vi "CenterFinder.vi"() -> ()   [LabVIEW 2016]
uses:
  Control/ProcessCtl.ctl
  <vilib>/userdefined/High Color/IMAQdx.ctl
  <vilib>/vision/driver/NI_Vision_Acquisition_Software.lvlib
  <vilib>/vision/NI_Vision_Development_Module.lvlib
panel:
  out "Array":T1(array[cluster])
  out "output cluster":cluster{"X":dbl, "Y":dbl, "Z":dbl}
  out "1":bool[](array[boolean])
  in  "Enum":enum16{"B2T", "L2R", "R2L", "T2B"}(ring)=enum."R2L"
  in  "Delete":bool
  in  "Retake":bool
  in  "Next":bool
  in  "Process":bool
  in  "Acquire":bool
  in  "stop":bool
  out "Image":T2(plugin-control)
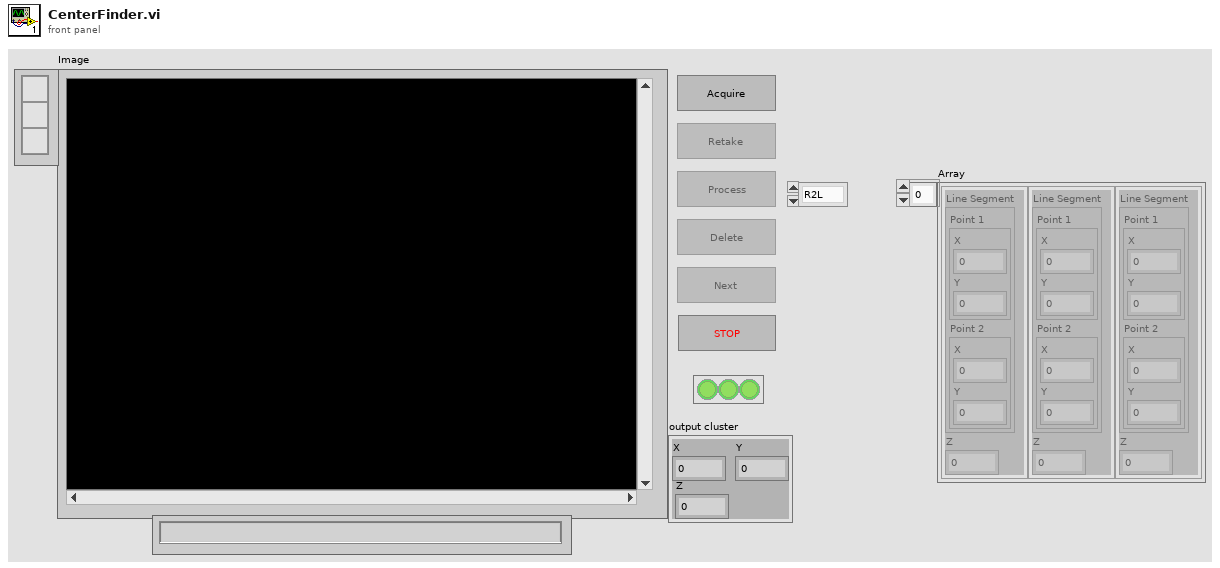
[diagram p1: front panel]
types:
  T1 = cluster{"Line Segment":cluster{"Point 1":cluster{"X":sgl, "Y":sgl}, "Point 2":cluster{"X":sgl, "Y":sgl}}, "Z":dbl}[]
  T2 = typedef "IMAQ Image.ctl" = refnum<image>
  T3 = typedef "IMAQdx.ctl" = refnum<k21>
  T4 = typedef "ProcessCtl.ctl" = enum16{"Idle", "Acquire", "Process", "Abort", "Initialize", "Wait"}
  T5 = enum8{"Enabled", "Disabled", "Disabled and Grayed Out"}
  T6 = cluster{"Line Segment":cluster{"Point 1":cluster{"X":sgl, "Y":sgl}, "Point 2":cluster{"X":sgl, "Y":sgl}}, "Z":dbl}
  T7 = cluster{"Edge Polarity":u16, "Kernel Size":u32, "Width":u32, "Minimum Edge Strength":dbl, "Interpolation Type":u16, "Data Processing Method":u16}
  T8 = typedef "Image Type" = u32
  T9 = typedef "IMAQ Line" = cluster{"Start X":i32, "Start Y":i32, "End X":i32, "End Y":i32}
  T10 = typedef "ROI Descriptor" = cluster{"Global Rectangle":i32[], "Contours":cluster{"ID":enum32{"External", "Internal"}, "Type":u32, "Coordinates":i32[]}[]}
  T11 = typedef "Edge New.ctl" = cluster{"Location (Pixel)":cluster{"X":sgl, "Y":sgl}, "Location (Real-World)":cluster{"X":sgl, "Y":sgl}, "Distance (Pixel)":dbl, "Distance (Real-World)":dbl, "Strength":dbl, "Noise":dbl, "Rising?":bool}
  T12 = cluster{"Point 1":cluster{"X":sgl, "Y":sgl}, "Point 2":cluster{"X":sgl, "Y":sgl}}
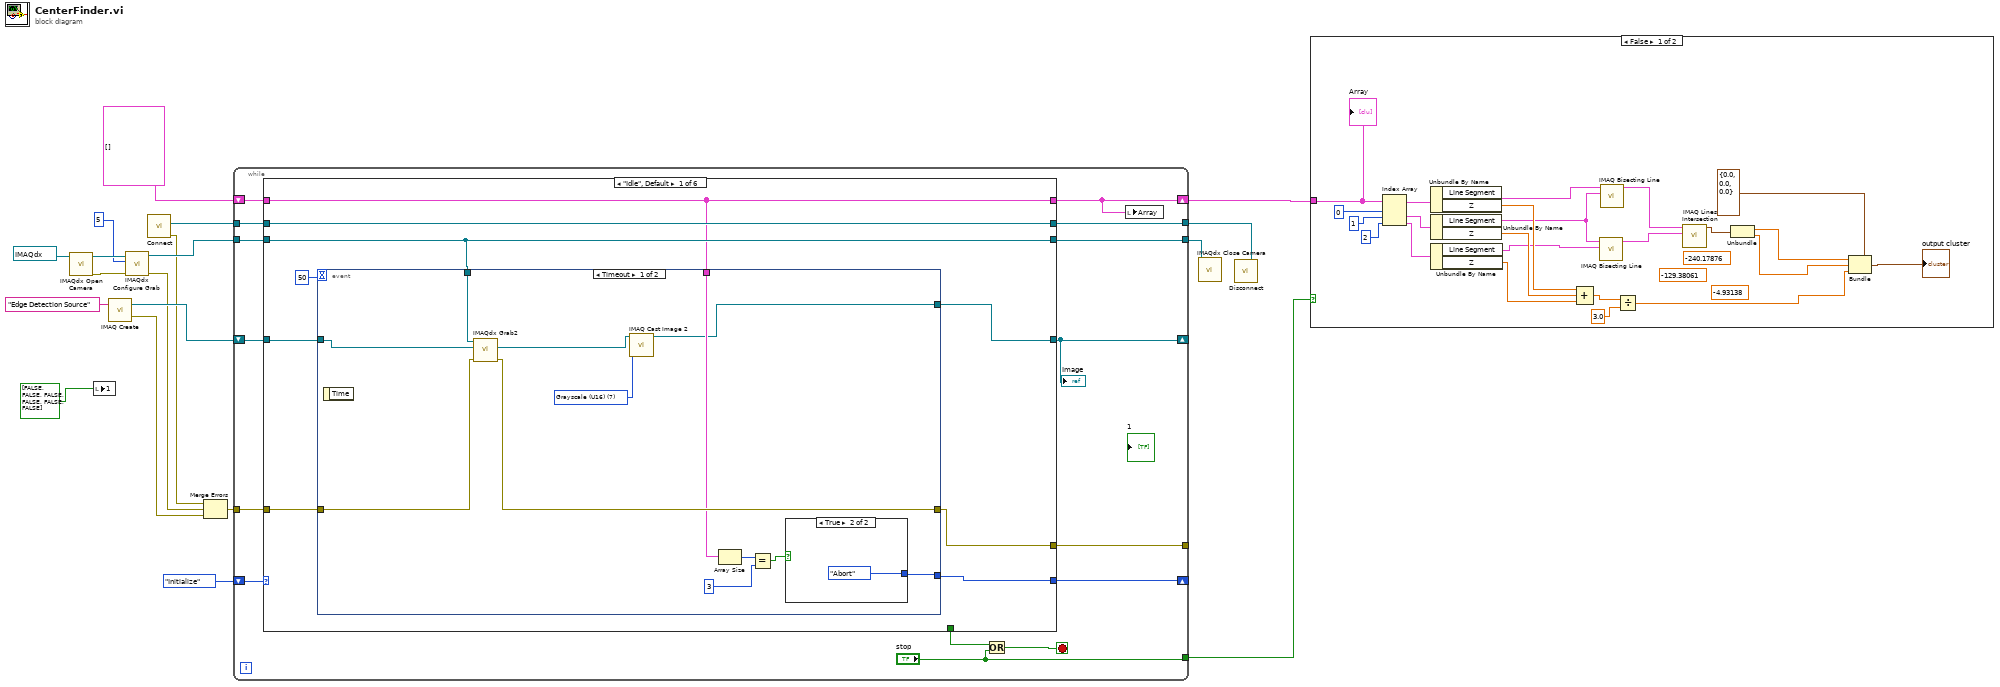
[diagram p0: block diagram]
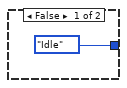
[diagram p3: hidden frame]
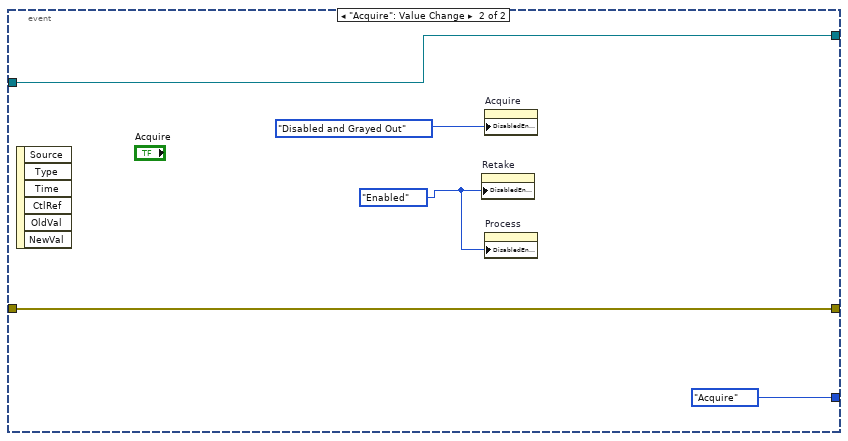
[diagram p4: hidden frame]
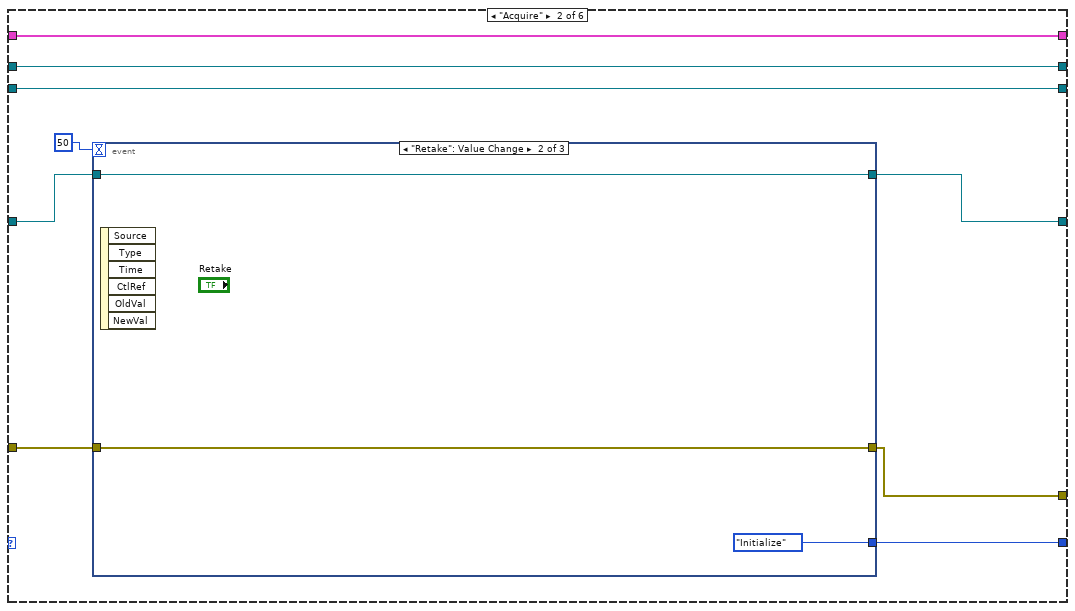
[diagram p5: hidden frame]
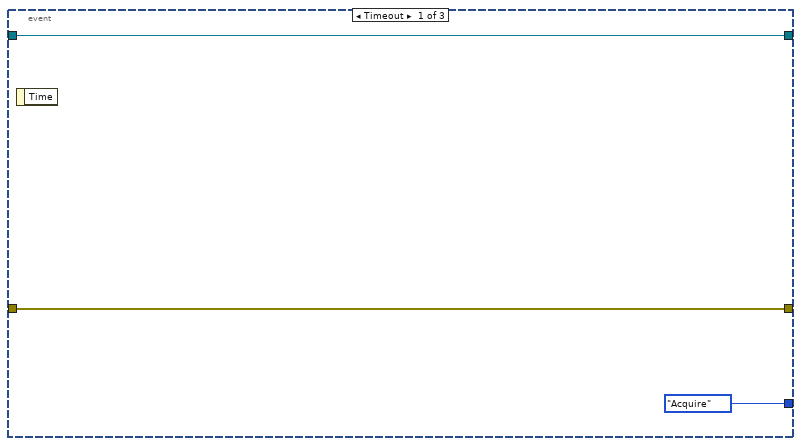
[diagram p6: hidden frame]
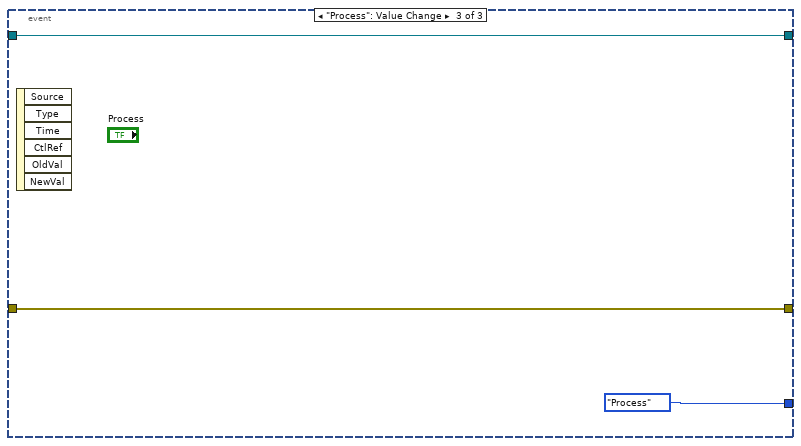
[diagram p7: hidden frame]
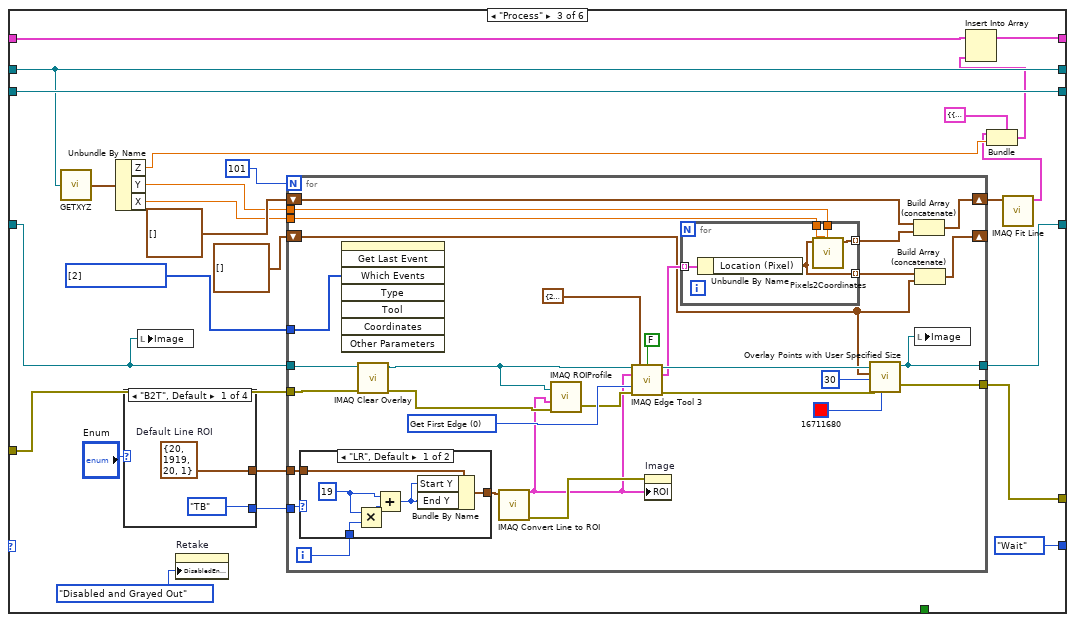
[diagram p8: hidden frame]
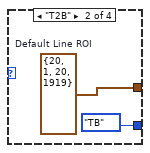
[diagram p9: hidden frame]
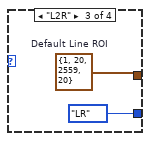
[diagram p10: hidden frame]
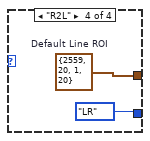
[diagram p11: hidden frame]
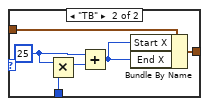
[diagram p12: hidden frame]
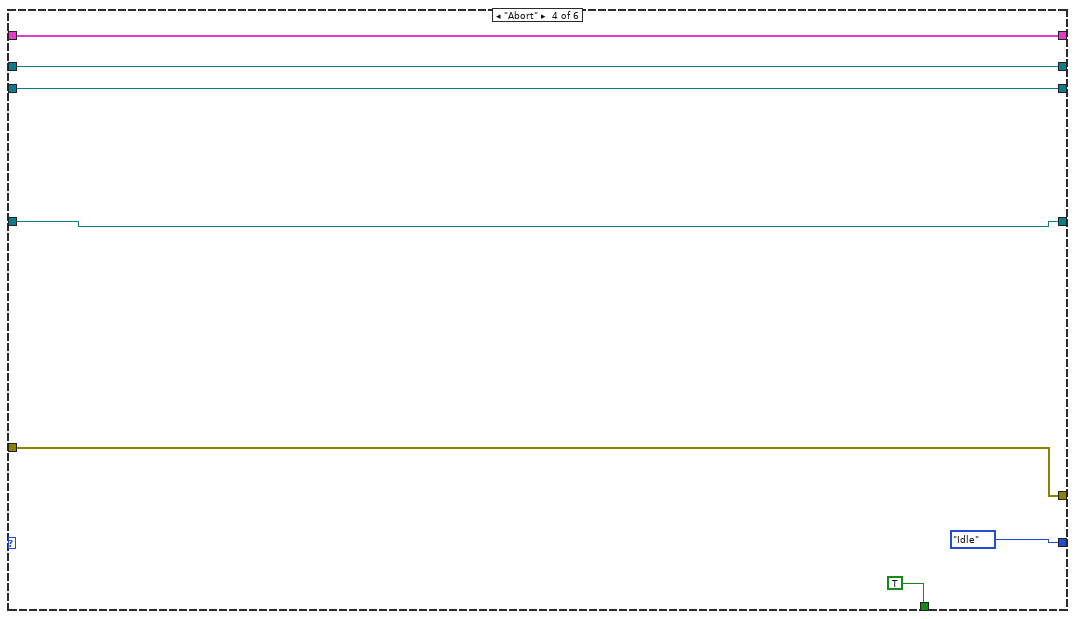
[diagram p13: hidden frame]
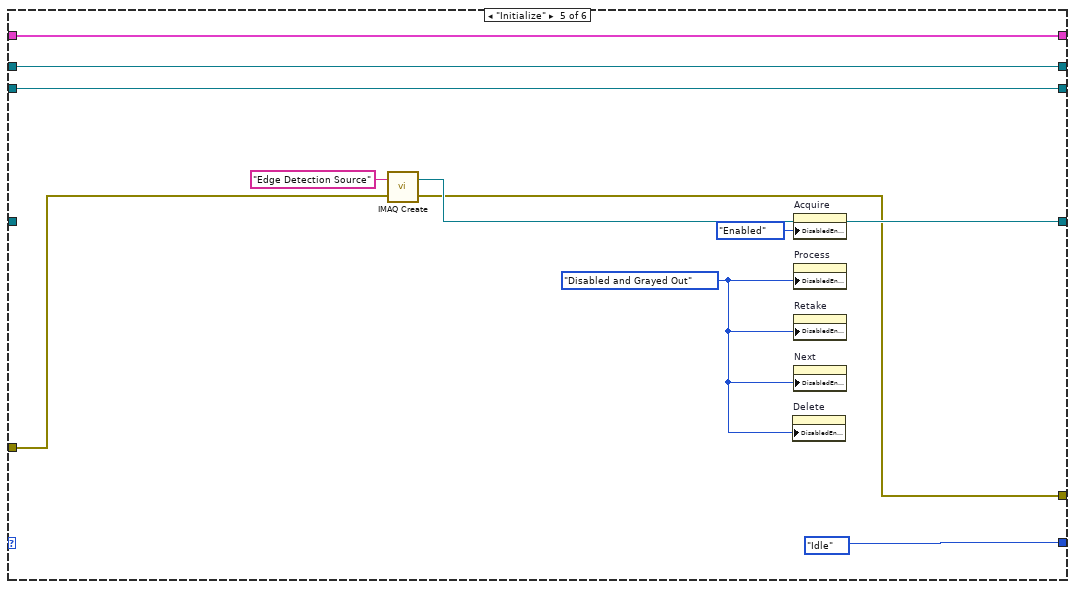
[diagram p14: hidden frame]
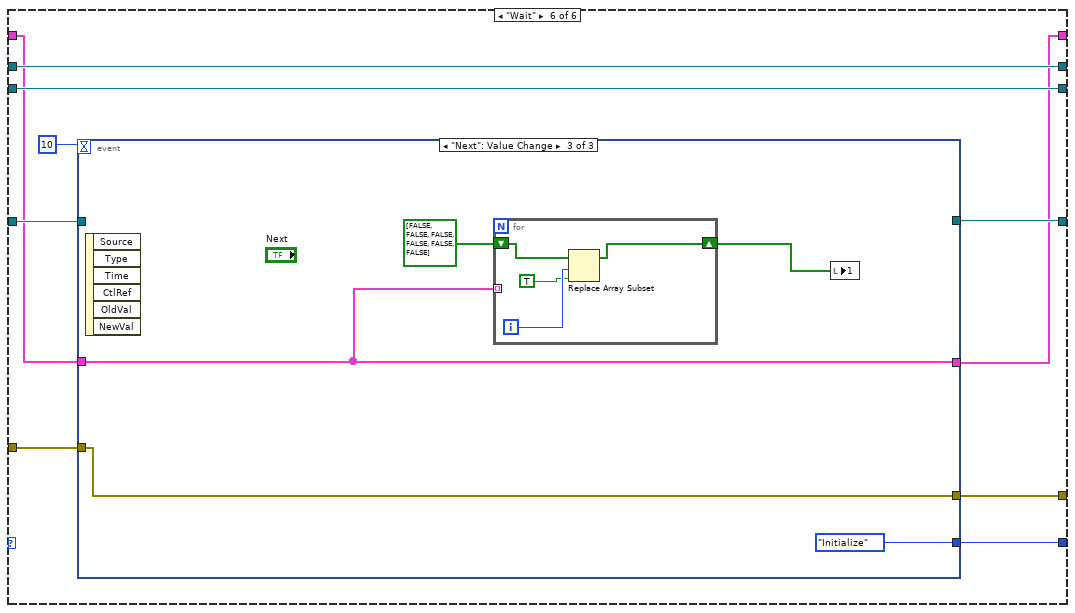
[diagram p15: hidden frame]
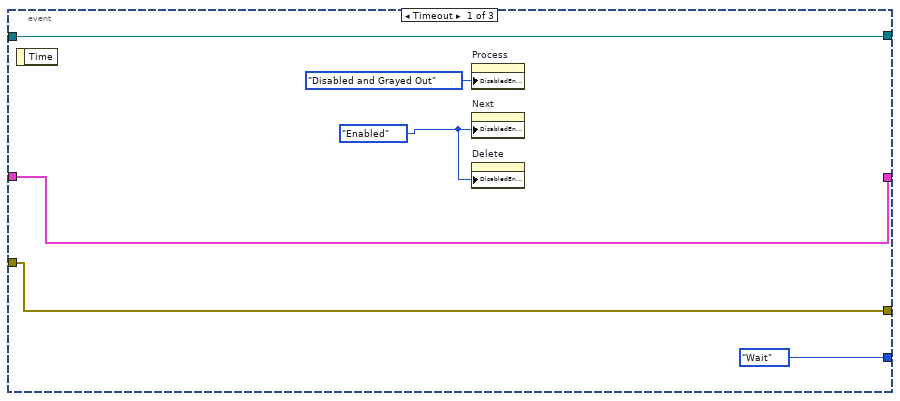
[diagram p16: hidden frame]
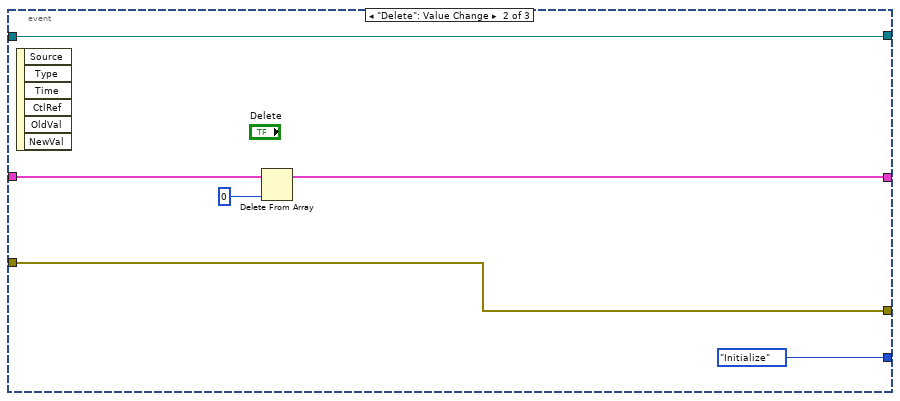
[diagram p17: hidden frame]
diagram:
  n1 = call <vilib>:"IMAQdx Open Camera.vi"("Session In"=T3 "cam0") -> ("error out"=w16:errorcluster, "Session Out"=w17:T3)  [unwired: 9 in]
  n2 = local write "1"(bool[] [FALSE, FALSE, FALSE, FALSE, FALSE, FALSE] ("1 2")) -> ()
  n3 = call "IMAQ Create"("Image Name"="Edge Detection Source") -> ("New Image"=w14:T2, "error out"=w7:errorcluster)  [unwired: 4 in]
  n4 = call <vilib>:"IMAQdx Configure Grab.vi"("error in"=w16, "Number of Buffers"=u32 5, "Session In"=w17) -> ("error out"=w8:errorcluster, "Session Out"=w18:T3)  [unwired: 7 in]
  n5 = call "Connect.vi"() -> ("error out"=w9:errorcluster, "controller"=w11:refnum<k24>)  [unwired: 10 in]
  n6 = Merge Errors(w9, w8, w7) -> (w6:errorcluster)
  n7 = while {
    tunnel: w18 -> [w25]
    tunnel: [w24] -> w12
    shift-right: [w31] -> _
    shift-left: w14 -> [w29]
    tunnel: w11 -> [w27]
    tunnel: [w26] -> w10
    tunnel: w6 -> [w34]
    shift-right: [w32] -> _
    shift-left: ProcessCtl."Initialize" -> [w33]
    tunnel: [w30] -> _
    shift-right: [w21] -> w2
    shift-left: T1 [] -> [w28]
    tunnel: ["stop"] -> w1
    stop <- w22 stop-if-true
    n8 = case shown="\"Idle\", Default" w33 {
      tunnel: w34 -> [w43 w67 w104 w161 w173 w179]
      tunnel: [w39 w68 ProcessCtl."Wait" ProcessCtl."Idle" ProcessCtl."Idle" w185] -> w32
      tunnel: w29 -> [w42 w71 w86 w164 _ w187]
      tunnel: [w41 w70 w96 w164 w174 w186] -> w31
      tunnel: [w38 w66 w90 w161 w172 w180] -> w30
      tunnel: w28 -> [w35 w65 w92 w167 w171 w182]
      tunnel: [w35 w65 w91 w167 w171 w181] -> w21
      tunnel: w27 -> [w37 w64 w93 w166 w170 w184]
      tunnel: [w37 w64 w93 w166 w170 w184] -> w26
      tunnel: w25 -> [w36 w63 w94 w165 w169 w183]
      tunnel: [w36 w63 w94 w165 w169 w183] -> w24
      tunnel: [_ _ _ TRUE _ _] -> w23
      frame "Idle", Default {
        n9 = event shown="[0] Timeout" {
          selector: _ -> [_ _]
          dyn-events: _ -> [_ _]
          timeout: 50 -> [_ _]
          tunnel: w43 -> [w55 w58]
          tunnel: w42 -> [w54 w60]
          tunnel: w36 -> [w53 _]
          tunnel: [w45 w60] -> w41
          tunnel: [w51 ProcessCtl."Acquire"] -> w39
          tunnel: [w52 w58] -> w38
          tunnel: w35 -> [w50 _]
          event Timeout {
            w46 = T8 7 items=["Grayscale (U8)", "Grayscale (I16)", "Grayscale (SGL)", "Complex (CSG)", "RGB (U32)", "HSL (U32)", "RGB (U64)", "Grayscale (U16)"] ("Image Type")
            n10 = event-data() -> ()  [unwired: 1 in, 1 out]
            n11 = call <vilib>:"IMAQdx Grab2.vi"("error in"=w55, "Image In"=w54, "Session In"=w53) -> ("error out"=w52:errorcluster, "Image Out"=w44:T2)  [unwired: 5 in, 2 out]
            n12 = call "IMAQ Cast Image 2"("Image Src"=w44, "Image Type"=w46) -> ("Image Dst Out"=w45:T2)  [unwired: 12 in, 1 out]
            n13 = Array Size(array=w50) -> (size(s)=w49:i32)
            n14 = Equal?(x=w49, y=3) -> (x = y?=w47:bool)
            n15 = case shown="True" w47 {
              tunnel: [ProcessCtl."Idle" ProcessCtl."Abort"] -> w51
              frame False {
              }
              frame True {
              }
            }
          }
          event "Acquire": Value Change {
            w59 = T5."Enabled" ("Disabled")
            n16 = event-data() -> ()  [unwired: 1 in, 6 out]
            n17 = property on="Retake" class="Bool"("DisabledEnum"=w59) -> ()  [unwired: 2 in, 2 out]
            n18 = property on="Acquire" class="Bool"("DisabledEnum"=T5."Disabled and Grayed Out" ("Disabled")) -> ()  [unwired: 2 in, 2 out]
            n19 = property on="Process" class="Bool"("DisabledEnum"=w59) -> ()  [unwired: 2 in, 2 out]
          }
        }
      }
      frame "Acquire" {
        n20 = event shown="[1] \"Retake\": Value Change" {
          selector: _ -> [_ _ _]
          dyn-events: _ -> [_ _ _]
          timeout: 50 -> [_ _ _]
          tunnel: w71 -> [w74 w75 w78]
          tunnel: [w74 w75 w78] -> w70
          tunnel: [ProcessCtl."Acquire" ProcessCtl."Initialize" ProcessCtl."Process"] -> w68
          tunnel: w67 -> [w72 w76 w79]
          tunnel: [w72 w76 w79] -> w66
          event Timeout {
            n21 = event-data() -> ()  [unwired: 1 in, 1 out]
          }
          event "Retake": Value Change {
            n22 = event-data() -> ()  [unwired: 1 in, 6 out]
          }
          event "Process": Value Change {
            n23 = event-data() -> ()  [unwired: 1 in, 6 out]
          }
        }
      }
      frame "Process" {
        w105 = i32[] [2] items=["No  event", "Click event", "Draw event", "Move event", "Size event", "Scroll event", "Activate event", "Close event", "Double click event"] ("Events list (all)")
        n24 = call "GETXYZ.vi"(".NET Refnum in"=w93) -> ("XYZ"=w99:cluster{"X":dbl, "Y":dbl, "Z":dbl})
        n25 = Unbundle By Name(w99) -> ("Z"=w83:dbl, "Y"=w98:dbl, "X"=w97:dbl)
        n26 = case shown="\"B2T\", Default" "Enum" {
          tunnel: [w107 w109 w110 w112] -> w102
          tunnel: [enum16{"LR", "TB"}."TB" enum16{"LR", "TB"}."TB" enum16{"LR", "TB"}."LR" enum16{"LR", "TB"}."LR"] -> w87
          frame "B2T", Default {
            w107 = T9 {"Start X"=20, "Start Y"=1919, "End X"=20, "End Y"=1}  # Default Line ROI
          }
          frame "T2B" {
            w109 = T9 {"Start X"=20, "Start Y"=1, "End X"=20, "End Y"=1919}  # Default Line ROI
          }
          frame "L2R" {
            w110 = T9 {"Start X"=1, "Start Y"=20, "End X"=2559, "End Y"=20}  # Default Line ROI
          }
          frame "R2L" {
            w112 = T9 {"Start X"=2559, "Start Y"=20, "End X"=1, "End Y"=20}  # Default Line ROI
          }
        }
        n27 = local write "Image"(w86) -> ()
        n28 = property on="Retake" class="Bool"("DisabledEnum"=T5."Disabled and Grayed Out" ("Disabled")) -> ()  [unwired: 2 in, 2 out]
        n29 = for {
          N: 101 -> [_]
          tunnel: w86 -> [w122]
          tunnel: w104 -> [w141]
          shift-right: [w132] -> w100
          shift-left: cluster{"X":sgl, "Y":sgl}[] [] -> [w134]
          tunnel: w105 -> [w126]
          tunnel: [w117] -> w96
          tunnel: [w131] -> w90
          tunnel: w102 -> [w129]
          tunnel: w98 -> [w128]
          tunnel: w97 -> [w127]
          tunnel: w87 -> [w124]
          shift-right: [w116] -> _
          shift-left: cluster{"X":sgl, "Y":sgl}[] [] -> [w114]
          i -> [w143]
          w140 = u16 0 items=["Get First Edge", "Get First + Last Edge", "Get All Edges", "Get Best Edge"] ("Process")
          n30 = case shown="\"LR\", Default" w124 {
            tunnel: w143 -> [w147 w155]
            tunnel: [w149 w151] -> w142
            tunnel: w129 -> [w148 w150]
            frame "LR", Default {
              w144 = 19
              n31 = Multiply(x=w144, y=w147) -> (x*y=w145:i32)
              n32 = Add(x=w144, y=w145) -> (x+y=w146:i32)
              n33 = Bundle By Name(cluster=w148, "Start Y"=w146, "End Y"=w146) -> (w149:T9)
            }
            frame "TB" {
              w153 = 25
              n34 = Multiply(x=w153, y=w155) -> (x*y=w154:i32)
              n35 = Add(x=w153, y=w154) -> (x+y=w152:i32)
              n36 = Bundle By Name(cluster=w150, "Start X"=w152, "End X"=w152) -> (w151:T9)
            }
          }
          n37 = invoke on="Image" class="ImageControl" method="Get Last Event"("Which Events"=w126) -> ()  [unwired: 7 in, 8 out]
          n38 = call "IMAQ Clear Overlay"("error in (no error)"=w141, "Image"=w122) -> ("error out"=w120:errorcluster, "Image Out"=w118:T2)  [unwired: 8 in]
          n39 = call "IMAQ Convert Line to ROI"("Line"=w142) -> ("error out"=w125:errorcluster, "ROI Descriptor"=w119:T10)  [unwired: 8 in]
          n40 = call "IMAQ ROIProfile"("error in (no error)"=w120, "ROI Descriptor"=w119, "Image"=w118) -> ("error out"=w121:errorcluster)  [unwired: 1 in, 4 out]
          n41 = call "IMAQ Edge Tool 3"("Image"=w118, "Edge Options"=T7 {"Edge Polarity"=2, "Kernel Size"=37, "Width"=5, "Minimum Edge Strength"=10.0, "Interpolation Type"=0, "Data Processing Method"=1}, "Optimized Mode"=FALSE, "ROI Descriptor"=w119, "Process"=w140, "error in (no error)"=w121) -> ("Image (duplicate)"=w137:T2, "Edge Information"=w123:T11[], "error out"=w136:errorcluster)  [unwired: 5 in, 2 out]
          n42 = property on="Image" class="ImageControl"(error in=w125, "ROI"=w119) -> ()  [unwired: 1 in, 2 out]
          n43 = for {
            tunnel: w123 -> [w160] mode=indexing
            tunnel: [w159] -> w133 mode=indexing
            tunnel: w128 -> [w158]
            tunnel: w127 -> [w157]
            tunnel: [w156] -> w115 mode=indexing
            n44 = Unbundle By Name(w160) -> ("Location (Pixel)"=w156:cluster{"X":sgl, "Y":sgl})
            n45 = call "Pixels2Coordinates.vi"("Y"=w158, "X"=w157, "Location (Pixel)"=w156) -> ("output cluster"=w159:cluster{"X":sgl, "Y":sgl})  [unwired: 8 in]
          }
          n46 = call "Overlay Points with User Specified Size.vi"("Color"=u32 16711680, "error in"=w136, "Point Diameter (5)"=30, "Points"=w114, "Image In"=w137) -> ("error out"=w131:errorcluster, "Image Out"=w117:T2)  [unwired: 5 in]
          n47 = Build Array (concatenate)(w134, w133) -> (w132:cluster{"X":sgl, "Y":sgl}[])
          n48 = Build Array (concatenate)(w115, w114) -> (w116:cluster{"X":sgl, "Y":sgl}[])
          n49 = local write "Image"(w117) -> ()
        }
        n50 = call "IMAQ Fit Line"("Points"=w100) -> ("Line Segment"=w82:T12)  [unwired: 5 in, 5 out]
        n51 = Bundle(cluster=T6 {"Line Segment"={"Point 1"={"X"=0.0, "Y"=0.0}, "Point 2"={"X"=0.0, "Y"=0.0}}, "Z"=0.0}, "Line Segment"=w82, "Z"=w83) -> (w81:T6)
        n52 = Insert Into Array(array=w92, new element=w81) -> (w91:T1)  [unwired: 1 in]
      }
      frame "Abort" {
      }
      frame "Initialize" {
        w168 = T5."Disabled and Grayed Out" ("Disabled")
        n53 = call "IMAQ Create"("Image Name"="Edge Detection Source", "error in (no error)"=w173) -> ("New Image"=w174:T2, "error out"=w172:errorcluster)  [unwired: 3 in]
        n54 = property on="Delete" class="Bool"("DisabledEnum"=w168) -> ()  [unwired: 2 in, 2 out]
        n55 = property on="Acquire" class="Bool"("DisabledEnum"=T5."Enabled" ("Disabled")) -> ()  [unwired: 2 in, 2 out]
        n56 = property on="Process" class="Bool"("DisabledEnum"=w168) -> ()  [unwired: 2 in, 2 out]
        n57 = property on="Retake" class="Bool"("DisabledEnum"=w168) -> ()  [unwired: 2 in, 2 out]
        n58 = property on="Next" class="Bool"("DisabledEnum"=w168) -> ()  [unwired: 2 in, 2 out]
      }
      frame "Wait" {
        n59 = event shown="[2] \"Next\": Value Change" {
          selector: _ -> [_ _ _]
          dyn-events: _ -> [_ _ _]
          timeout: 10 -> [_ _ _]
          tunnel: w187 -> [w193 w196 _]
          tunnel: [w193 w196 _] -> w186
          tunnel: [ProcessCtl."Wait" ProcessCtl."Initialize" ProcessCtl."Initialize"] -> w185
          tunnel: w182 -> [w191 w199 w202]
          tunnel: [w191 w198 w202] -> w181
          tunnel: [w190 w194 w203] -> w180
          tunnel: w179 -> [w190 w194 w203]
          event Timeout {
            w188 = T5."Enabled" ("Disabled")
            n60 = event-data() -> ()  [unwired: 1 in, 1 out]
            n61 = property on="Process" class="Bool"("DisabledEnum"=T5."Disabled and Grayed Out" ("Disabled")) -> ()  [unwired: 2 in, 2 out]
            n62 = property on="Next" class="Bool"("DisabledEnum"=w188) -> ()  [unwired: 2 in, 2 out]
            n63 = property on="Delete" class="Bool"("DisabledEnum"=w188) -> ()  [unwired: 2 in, 2 out]
          }
          event "Delete": Value Change {
            n64 = event-data() -> ()  [unwired: 1 in, 6 out]
            n65 = Delete From Array(array=w199, index=0) -> (array with subset deleted=w198:T1)  [unwired: 1 in, 1 out]
          }
          event "Next": Value Change {
            n66 = event-data() -> ()  [unwired: 1 in, 6 out]
            n67 = for {
              tunnel: w202 -> [_] mode=indexing
              shift-right: [w205] -> w200
              shift-left: bool[] [FALSE, FALSE, FALSE, FALSE, FALSE, FALSE] ("1 2") -> [w208]
              i -> [w207]
              n68 = Replace Array Subset(array=w208, new element=TRUE, index=w207) -> (w205:bool[])
            }
            n69 = local write "1"(w200) -> ()
          }
        }
      }
    }
    "Image" <- w31
    n70 = Or(x=w23, y="stop") -> (x .or. y?=w22:bool)
    n71 = local write "Array"(w21) -> ()
  }
  n72 = call <vilib>:"IMAQdx Close Camera.vi"("Session In"=w12) -> ()  [unwired: 10 in, 1 out]
  n73 = call "Disconnect.vi"("controller"=w10) -> ()  [unwired: 10 in, 1 out]
  n74 = case shown="False" w1 {
    tunnel: w2 -> [w231 _]
    frame False {
      (unwired) -4.93138
      (unwired) -129.38061
      (unwired) -240.17876
      n75 = Index Array(array=w231, index #1=0, index #2=1, index #3=2) -> (element #1=w227:T6, element #2=w226:T6, element #3=w225:T6)
      n76 = Unbundle By Name(w227) -> ("Line Segment"=w214:T12, "Z"=w222:dbl)
      n77 = Unbundle By Name(w226) -> ("Line Segment"=w212:T12, "Z"=w221:dbl)
      n78 = Unbundle By Name(w225) -> ("Line Segment"=w213:T12, "Z"=w220:dbl)
      n79 = Compound Arithmetic op=ADD(w222, w221, w220) -> (w219:dbl)
      n80 = call "IMAQ Bisecting Line"("Line 2"=w213, "Line 1"=w212) -> ("Bisecting Line"=w223:T12)  [unwired: 8 in, 1 out]
      n81 = call "IMAQ Bisecting Line"("Line 2"=w212, "Line 1"=w214) -> ("Bisecting Line"=w224:T12)  [unwired: 8 in, 1 out]
      n82 = Divide(x=w219, y=3.0) -> (x/y=w210:dbl)
      n83 = call "IMAQ Lines Intersection"("Line 2"=w223, "Line 1"=w224) -> ("Intersection Point"=w217:cluster{"X":sgl, "Y":sgl})  [unwired: 7 in, 2 out]
      n84 = Unbundle(w217) -> ("X"=w209:sgl, "Y"=w211:sgl)
      n85 = Bundle(cluster=cluster{"X":dbl, "Y":dbl, "Z":dbl} {"X"=0.0, "Y"=0.0, "Z"=0.0}, "X"=w209, "Y"=w211, "Z"=w210) -> (→"output cluster":cluster{"X":dbl, "Y":dbl, "Z":dbl})
      "Array" <- w231
    }
    frame True {
    }
  }
